vi "ParseIPControl.vi"(1 "data out":string) -> (2 "dstId":u16, 3 "srcId":u16, 4 "panId":u16, 5 "Bytes Read":i32)   [LabVIEW 2010]
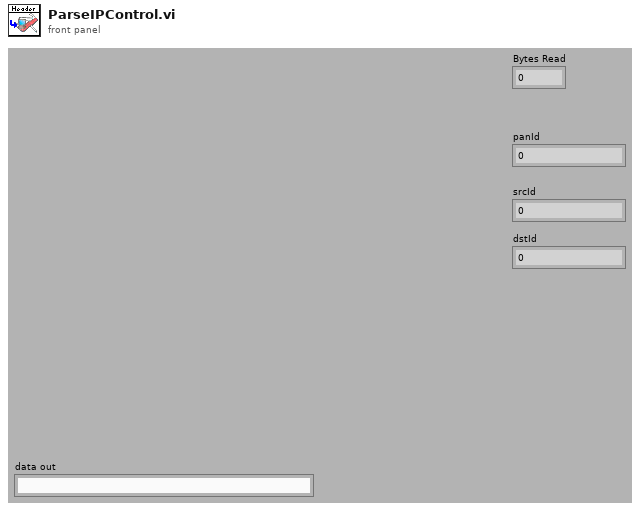
[diagram p1: front panel]
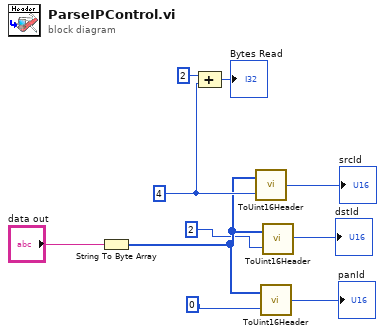
[diagram p0: block diagram]
diagram:
  w4 = 4 ("index")
  n1 = String To Byte Array(string="data out") -> (unsigned byte array=w2:u8[])
  n2 = Compound Arithmetic op=unknown(2 ("value"), w4) -> (→"Bytes Read":i32)
  n3 = call "ToUint16Header.vi"("index"=w4, "array"=w2) -> ("sp float"=→"srcId":u16)
  n4 = call "ToUint16Header.vi"("index"=0, "array"=w2) -> ("sp float"=→"panId":u16)
  n5 = call "ToUint16Header.vi"("index"=2, "array"=w2) -> ("sp float"=→"dstId":u16)
